vi "ma_Check Sampling Info.vi"(4 "error in (no error)":errorcluster, 7 "sampling info":cluster{"Fs":dbl, "#s":dbl}={"Fs"=1000.0, "#s"=1000.0} {"Fs" format="%.1p"}) -> (0 "error out":errorcluster, 3 "sampling info is ok":bool)   [LabVIEW 2020, in "NI_MABase.lvlib"]
uses:
  NI_MABase.lvlib
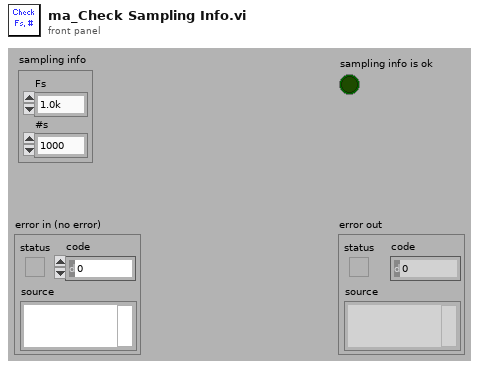
[diagram p1: front panel]
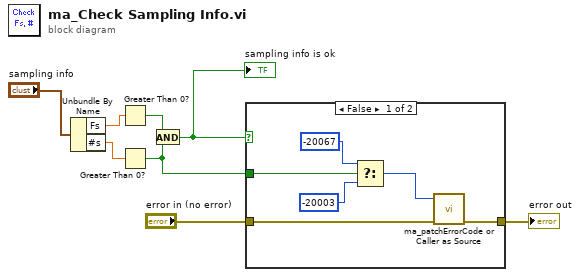
[diagram p0: block diagram]
diagram:
  n1 = Unbundle By Name("sampling info") -> ("Fs"=w6:dbl, "#s"=w5:dbl)
  n2 = Greater Than 0?(x=w6) -> (x > 0?=w8:bool)
  n3 = Greater Than 0?(x=w5) -> (x > 0?=w4:bool)
  n4 = And(x=w8, y=w4) -> (x .and. y?=w3:bool)
  "sampling info is ok" <- w3
  n5 = case shown="False" w3 {
    tunnel: w4 -> [w11 _]
    tunnel: "error in (no error)" -> [w10 w15]
    tunnel: [w9 w15] -> w2
    frame False {
      n6 = Select(t=-20067 ("code"), s=w11, f=-20003 ("code")) -> (s? t:f=w12:i32)
      n7 = call "ma_patchErrorCode or Caller as Source.vi"("error in (no error)"=w10, "error code"=w12) -> ("error out"=w9:errorcluster)  [unwired: 9 in]
    }
    frame True {
    }
  }
  "error out" <- w2
